vi "PI Start WG.vi"(0 "System no.":i32=1 min=1 max=4 step=1, 1 "axis":string="xy", 2 "Generator":i8 min=0 max=2 step=1, 3 "Init DDL":i8 min=0 max=3 step=1, 4 "increment":i8 min=0 max=3 step=1, 5 "error in":errorcluster, 14 "saved data":i8 min=0 max=3 step=1) -> (19 "error out":errorcluster)   [LabVIEW 2011]
doc: "Sends command with or without trailing linefeed to selected system. \n\nValid for C-843, C-843.PM, C-844, C-848, C-865, C-880, C-880K005, E-516, E-710, E-816, F-206, M-8X0"
uses:
  <userlib>/E710_GCS_LabVIEW/Low Level/Communication.llb/Global1.vi
panel:
  out "String":string
  # "This vi sends a string w/o linefeed via the GPIB interface."
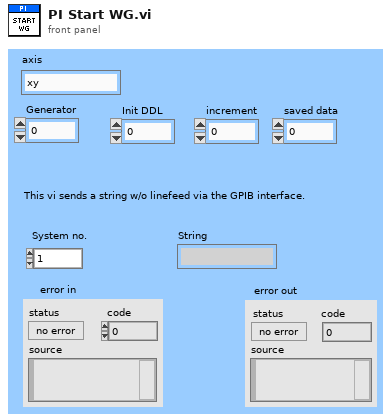
[diagram p1: front panel]
types:
  T1 = cluster{"RS232 Portnumber":u16, "Timeout":u32, "RS232 Baud rate":u32, "Interface":u16, "GPIB Bus":i32, "GPIB Address":i32, "GPIB Mode":i32}[]
  T2 = cluster{"RS232 Portnumber":u16, "Timeout":u32, "RS232 Baud rate":u32, "Interface":u16, "GPIB Bus":i32, "GPIB Address":i32, "GPIB Mode":i32}
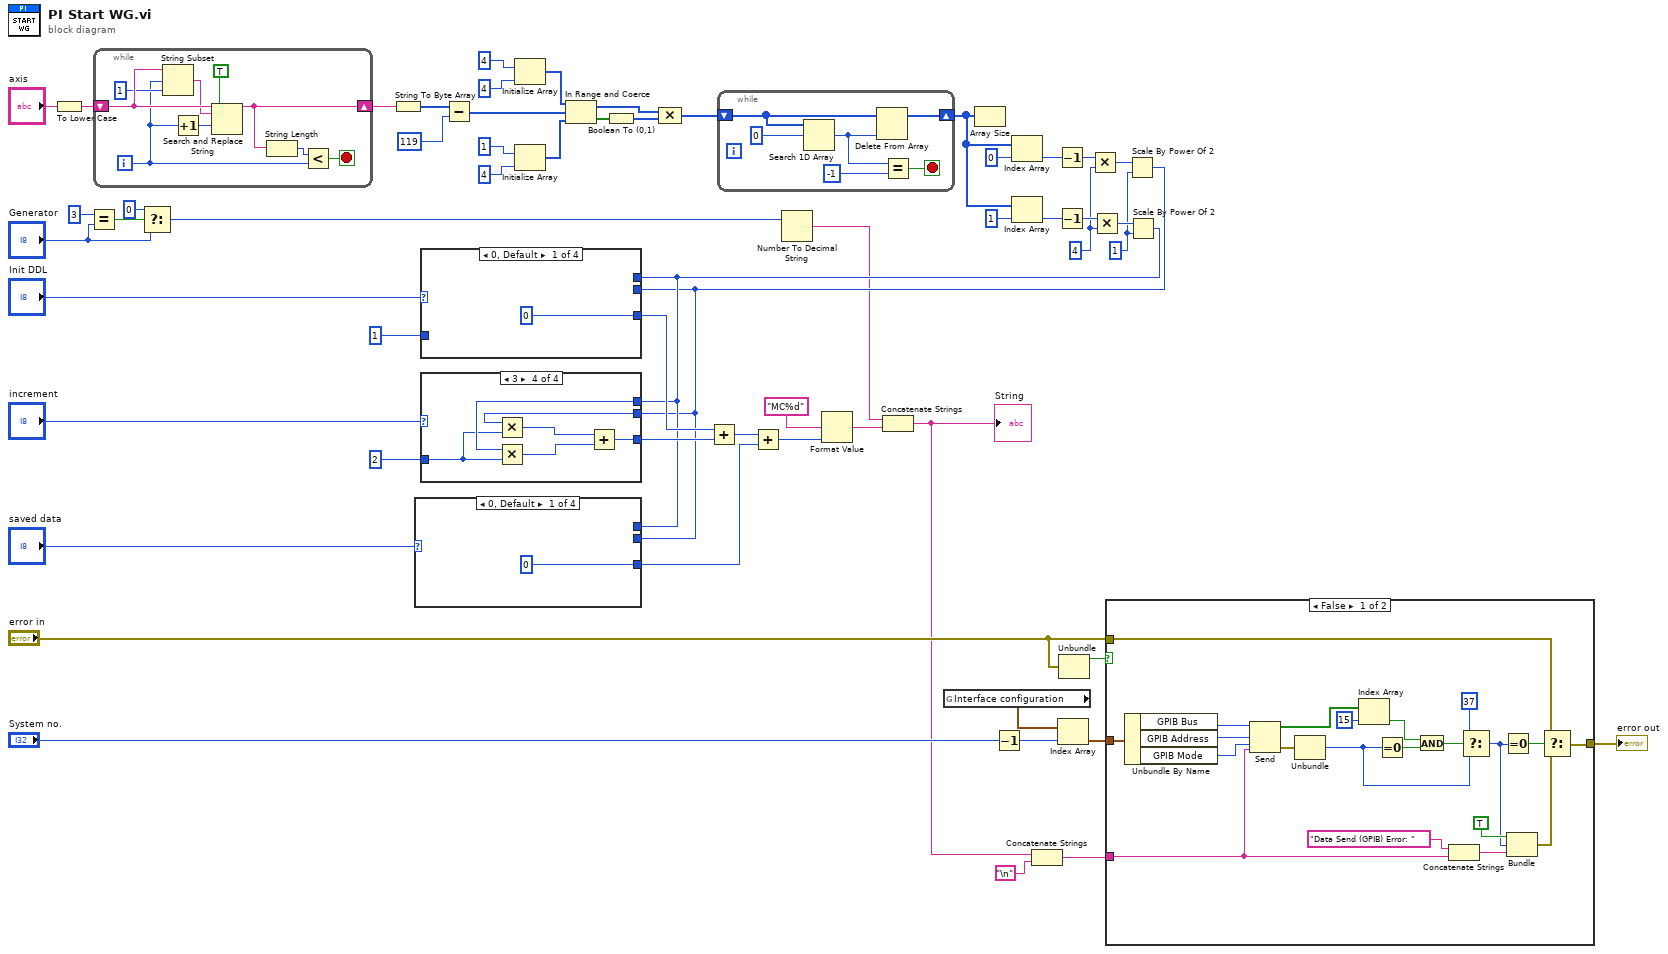
[diagram p0: block diagram]
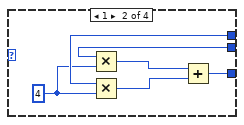
[diagram p2: hidden frame]
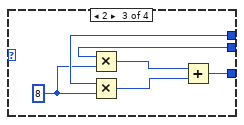
[diagram p3: hidden frame]
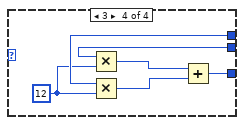
[diagram p4: hidden frame]
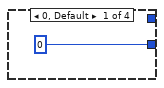
[diagram p5: hidden frame]
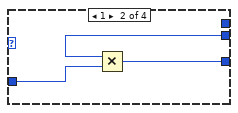
[diagram p6: hidden frame]
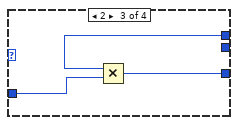
[diagram p7: hidden frame]
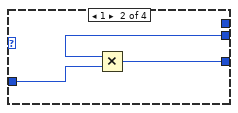
[diagram p8: hidden frame]
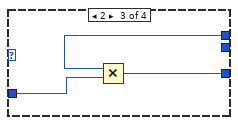
[diagram p9: hidden frame]
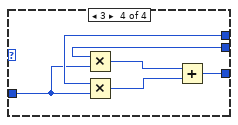
[diagram p10: hidden frame]
diagram:
  w22 = 1
  w23 = 4
  n1 = To Lower Case(string="axis") -> (all lower case string=w34:string)
  n2 = Equal?(x=3, y="Generator") -> (x = y?=w5:bool)
  n3 = while {
    shift-right: [w62] -> w39
    shift-left: w34 -> [w66]
    i -> [w58]
    stop <- w61 stop-if-true
    n4 = String Subset(string=w66, offset (0)=w58, length (rest)=1) -> (substring=w64:string)
    n5 = Increment(x=w58) -> (x+1=w59:i32)
    n6 = Search and Replace String(replace all?=TRUE, input string=w66, search string=w64, offset=w59) -> (result string=w62:string)  [unwired: 4 in, 3 out]
    n7 = String Length(string=w62) -> (length=w60:i32)
    n8 = Less?(x=w60, y=w58) -> (x < y?=w61:bool)
  }
  n9 = Select(t=0, s=w5, f="Generator") -> (s? t:f=w3:i32)
  n10 = String To Byte Array(string=w39) -> (unsigned byte array=w41:u8[])
  n11 = Subtract(x=w41, y=119) -> (x-y=w38:i32[])
  n12 = Initialize Array(4, 4) -> (w46:i32[])
  n13 = Initialize Array(1, 4) -> (w43:i32[])
  n14 = In Range and Coerce(upper limit=w46, x=w38, lower limit=w43) -> (coerced(x)=w35:i32[], In Range?=w42:bool[])
  n15 = Boolean To (0,1)(Boolean=w42) -> (0, 1=w36:i16[])
  n16 = Compound Arithmetic op=MULTIPLY(w35, w36) -> (w37:i32[])
  n17 = while {
    shift-right: [w69] -> w31
    shift-left: w37 -> [w67]
    stop <- w70 stop-if-true
    n18 = Search 1D Array(1D array=w67, element=0) -> (index of element=w71:i32)  [unwired: 1 in]
    n19 = Delete From Array(array=w67, index=w71) -> (array with subset deleted=w69:i32[])  [unwired: 1 in, 1 out]
    n20 = Equal?(x=w71, y=-1) -> (x = y?=w70:bool)
  }
  n21 = Number To Decimal String(number=w3) -> (decimal integer string=w6:string)  [unwired: 1 in]
  n22 = global read "Global1.vi" "Interface configuration"() -> (w53:T1)
  n23 = Array Size(array=w31) -> ()  [unwired: 1 out]
  n24 = Decrement(x="System no.") -> (x-1=w50:i32)
  n25 = Index Array(array=w31, index=0) -> (element=w30:i32)
  n26 = Index Array(array=w31, index=1) -> (element=w29:i32)
  n27 = Decrement(x=w30) -> (x-1=w27:i32)
  n28 = Decrement(x=w29) -> (x-1=w26:i32)
  n29 = Index Array(array=w53, index=w50) -> (element=w52:T2)
  n30 = Unbundle("error in") -> ("status"=w57:bool)  [unwired: 2 out]
  n31 = Multiply(x=w27, y=w23) -> (x*y=w25:i32)
  n32 = Multiply(x=w26, y=w23) -> (x*y=w24:i32)
  n33 = Scale By Power Of 2(n=w25, x=w22) -> (x*2^n=w13:i32)
  n34 = Scale By Power Of 2(n=w24, x=w22) -> (x*2^n=w14:i32)
  n35 = case shown="0, Default" "saved data" {
    tunnel: w13 -> [_ w75 w81 w87]
    tunnel: [0 w78 w84 w90] -> w11
    tunnel: w14 -> [_ w79 w85 w91]
    frame 0, Default {
    }
    frame 1 {
      w74 = 4
      n36 = Multiply(x=w75, y=w74) -> (x*y=w76:i32)
      n37 = Multiply(x=w79, y=w74) -> (x*y=w77:i32)
      n38 = Add(x=w76, y=w77) -> (x+y=w78:i32)
    }
    frame 2 {
      w80 = 8
      n39 = Multiply(x=w81, y=w80) -> (x*y=w82:i32)
      n40 = Multiply(x=w85, y=w80) -> (x*y=w83:i32)
      n41 = Add(x=w82, y=w83) -> (x+y=w84:i32)
    }
    frame 3 {
      w86 = 12
      n42 = Multiply(x=w87, y=w86) -> (x*y=w88:i32)
      n43 = Multiply(x=w91, y=w86) -> (x*y=w89:i32)
      n44 = Add(x=w88, y=w89) -> (x+y=w90:i32)
    }
  }
  n45 = case shown="0, Default" "Init DDL" {
    tunnel: w13 -> [_ w95 _ w99]
    tunnel: [0 w94 w98 w102] -> w18
    tunnel: w14 -> [_ _ w96 w104]
    tunnel: 1 -> [_ w93 w97 w103]
    frame 0, Default {
    }
    frame 1 {
      n46 = Multiply(x=w95, y=w93) -> (x*y=w94:i32)
    }
    frame 2 {
      n47 = Multiply(x=w96, y=w97) -> (x*y=w98:i32)
    }
    frame 3 {
      n48 = Multiply(x=w99, y=w103) -> (x*y=w100:i32)
      n49 = Multiply(x=w104, y=w103) -> (x*y=w101:i32)
      n50 = Add(x=w100, y=w101) -> (x+y=w102:i32)
    }
  }
  n51 = case shown="3" "increment" {
    tunnel: w13 -> [_ w108 _ w112]
    tunnel: [0 w107 w111 w115] -> w17
    tunnel: w14 -> [_ _ w109 w117]
    tunnel: 2 -> [_ w106 w110 w116]
    frame 0, Default {
    }
    frame 1 {
      n52 = Multiply(x=w108, y=w106) -> (x*y=w107:i32)
    }
    frame 2 {
      n53 = Multiply(x=w109, y=w110) -> (x*y=w111:i32)
    }
    frame 3 {
      n54 = Multiply(x=w112, y=w116) -> (x*y=w113:i32)
      n55 = Multiply(x=w117, y=w116) -> (x*y=w114:i32)
      n56 = Add(x=w113, y=w114) -> (x+y=w115:i32)
    }
  }
  n57 = Add(x=w18, y=w17) -> (x+y=w12:i32)
  n58 = Add(x=w12, y=w11) -> (x+y=w10:i32)
  n59 = Format Value(format string="MC%d", value (0)=w10) -> (output string=w7:string)  [unwired: 1 in]
  n60 = Concatenate Strings(w6, w7) -> (w8:string)
  "String" <- w8
  n61 = Concatenate Strings(w8, "\n") -> (w54:string)
  n62 = case shown="False" w57 {
    tunnel: [w121 w139] -> w55
    tunnel: "error in" -> [w123 w139]
    tunnel: w54 -> [w119 _]
    tunnel: w52 -> [w122 _]
    frame False {
      n63 = Unbundle By Name(w122) -> ("GPIB Bus"=w138:i32, "GPIB Address"=w137:i32, "GPIB Mode"=w136:i32)
      n64 = Send(0:w138, 2:w137, 3:w136, 5:w119) -> (6:w130:bool[], 8:w135:errorcluster)  [unwired: 1 in, 1 out]
      n65 = Unbundle(w135) -> ("code"=w128:i32)  [unwired: 2 out]
      n66 = Index Array(array=w130, index=15 ("Index")) -> (element=w129:bool)
      n67 = Equal To 0?(x=w128) -> (x = 0?=w131:bool)
      n68 = And(x=w129, y=w131) -> (x .and. y?=w133:bool)
      n69 = Concatenate Strings("Data Send (GPIB) Error: ", w119) -> (w118:string)
      n70 = Select(t=37, s=w133, f=w128) -> (s? t:f=w126:i32)
      n71 = Equal To 0?(x=w126) -> (x = 0?=w125:bool)
      n72 = Bundle(TRUE, "code"=w126, w118) -> (w124:cluster{bool, "code":i32, string})  [unwired: 1 in]
      n73 = Select(t=w123, s=w125, f=w124) -> (s? t:f=w121:errorcluster)
    }
    frame True {
      # "Error!"
    }
  }
  "error out" <- w55
